vi "Format number_123.vi"(1 "number":i32) -> (0 "String":string)   [LabVIEW 2016]
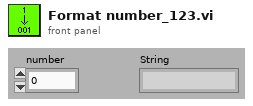
[diagram p1: front panel]
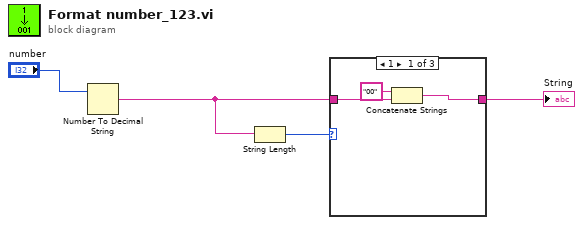
[diagram p0: block diagram]
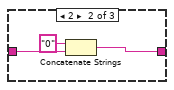
[diagram p2: hidden frame]
diagram:
  n1 = Number To Decimal String(number="number") -> (decimal integer string=w2:string)  [unwired: 1 out]
  n2 = String Length(string=w2) -> (length=w3:i32)
  n3 = case shown="1" w3 {
    tunnel: w2 -> [w7 w10 w11]
    tunnel: [w5 w9 w11] -> w1
    frame 1 {
      n4 = Concatenate Strings("00" ("string"), w7) -> (w5:string)
    }
    frame 2 {
      n5 = Concatenate Strings("0" ("string"), w10) -> (w9:string)
    }
    frame 3, Default {
    }
  }
  "String" <- w1
